vi "POST (Buffer).vi"(6 "timeout":i32=10000, 7 "output file":path, 8 "error in":errorcluster, 9 "buffer":string, 10 "url":string, 11 "session in":refnum<class "Session.lvclass">) -> (0 "error out":errorcluster, 1 "body":string, 2 "headers":string, 3 "session out":refnum<class "Session.lvclass">, 4 "status code":u32)   [LabVIEW 2019, in "NI_Advanced HTTP Client.lvlib" / "Session.lvclass"]
uses:
  Session.lvclass
  Session.lvclass/Session.ctl
  lvwebclient_32.dll
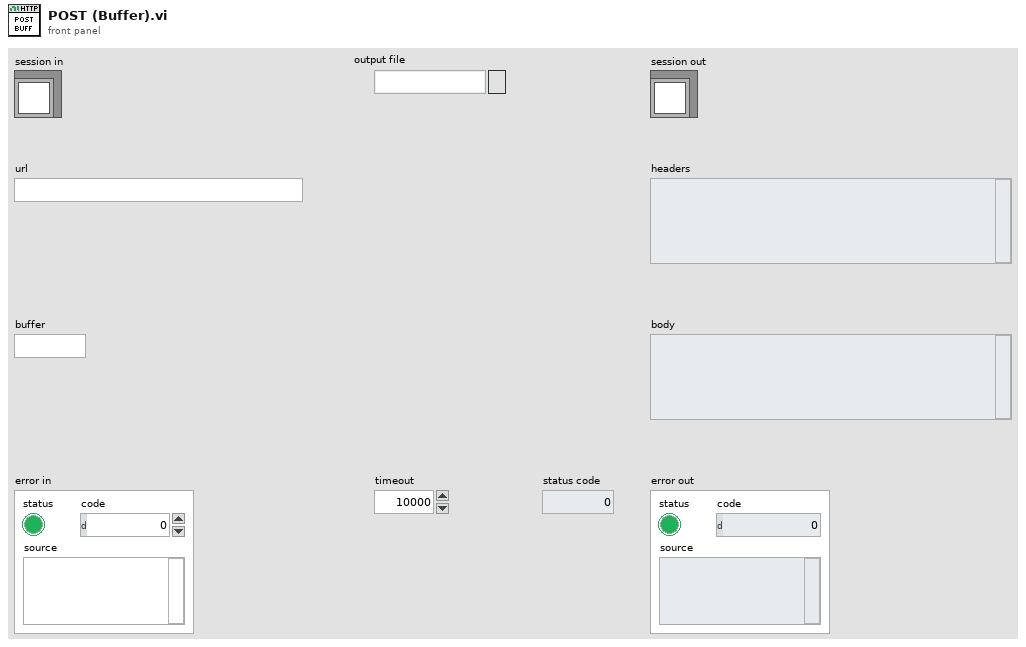
[diagram p1: front panel]
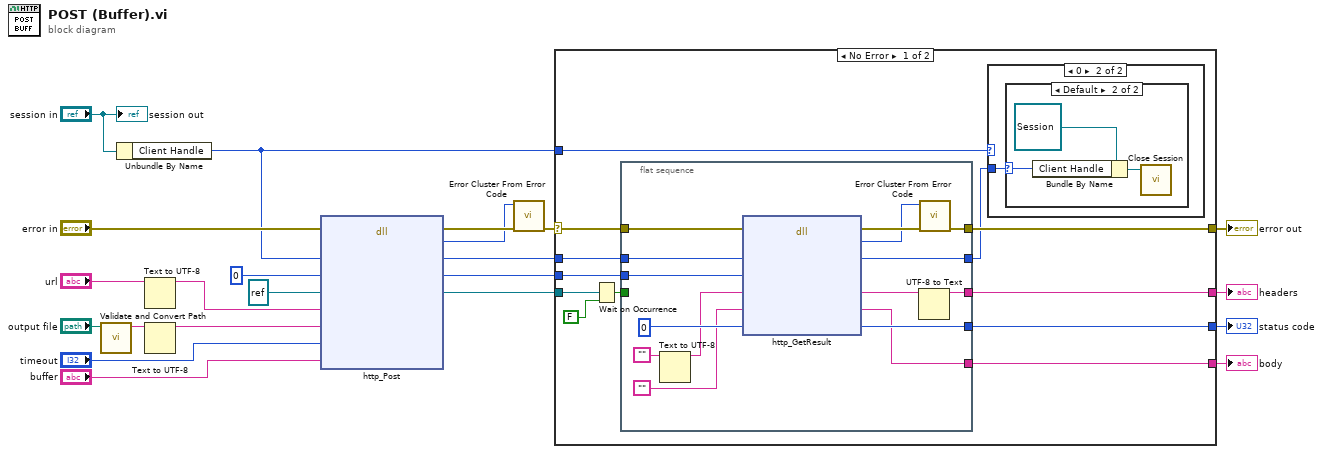
[diagram p0: block diagram]
diagram:
  n1 = call "Validate and Convert Path.vi"("path"="output file") -> ("validated path as string"=w14:string)  [unwired: 10 in]
  n2 = Unbundle By Name("session in") -> ("Client Handle"=w5:u32)
  n3 = Text to UTF-8(11:"url") -> (3:w3:string)  [unwired: 2 in, 1 out]
  n4 = Text to UTF-8(11:w14) -> (3:w2:string)  [unwired: 2 in, 1 out]
  n5 = dll-call lib="C:/Users/Localization Tester/Desktop/ni-adv-http-api/Advanced HTTP Client/lvwebclient_*.*" fn="http_Post"(error in="error in", "handle"=w5, "request"=u32 0, "completeOccurrence"=refnum<k4> refnum ("occurrence"), "url"=w3, "outPath"=w2, "timeout"="timeout", "postData"="buffer") -> (error out=w11:errorcluster, "return"=w10:i32, "handle"=w9:u32, "request"=w8:u32, "completeOccurrence"=w6:refnum<k4>)  [unwired: 6 in, 1 out]
  n6 = call <vilib>:"Error Cluster From Error Code.vi"("error in (no error)"=w11, "error code (0)"=w10) -> ("error out"=w22:errorcluster)  [unwired: 7 in]
  n7 = case shown="No Error" w22 {
    selector: w22 -> [w32 w54]
    tunnel: w6 -> [w34 _]
    tunnel: w9 -> [w31 _]
    tunnel: w8 -> [w30 _]
    tunnel: [w29 _] -> w19
    tunnel: [w28 _] -> w18
    tunnel: [w27 _] -> w17
    tunnel: [w26 w54] -> w16
    tunnel: w5 -> [w25 _]
    frame No Error {
      n8 = Wait on Occurrence(1:FALSE, 2:w34) -> (0:w33:bool)  [unwired: 1 in]
      n9 = flat-sequence {
        tunnel: w33 -> [_]
        tunnel: w32 -> [w53]
        tunnel: w31 -> [w52]
        tunnel: w30 -> [w51]
        tunnel: [w49] -> w29
        tunnel: [w44] -> w28
        tunnel: [w45] -> w27
        tunnel: [w43] -> w26
        tunnel: [w42] -> w24
        frame #0 {
          n10 = Text to UTF-8(11:"") -> (3:w40:string)  [unwired: 2 in, 1 out]
          n11 = dll-call lib="C:/Users/Localization Tester/Desktop/ni-adv-http-api/Advanced HTTP Client/lvwebclient_*.*" fn="http_GetResult"(error in=w53, "handle"=w52, "request"=w51, "returnHeader"=w40, "returnBody"="", "httpStatus"=u32 0) -> (error out=w48:errorcluster, "return"=w47:i32, "handle"=w42:u32, "returnHeader"=w46:string, "returnBody"=w45:string, "httpStatus"=w49:u32)  [unwired: 3 in, 1 out]
          n12 = UTF-8 to Text(11:w46) -> (3:w44:string)  [unwired: 2 in, 1 out]
          n13 = call <vilib>:"Error Cluster From Error Code.vi"("error in (no error)"=w48, "error code (0)"=w47) -> ("error out"=w43:errorcluster)  [unwired: 7 in]
        }
      }
      n14 = case shown="0" w25 {
        tunnel: w24 -> [_ w35]
        frame Default {
        }
        frame 0 {
          n15 = case shown="Default" w35 {
            selector: w35 -> [_ w38]
            frame 0 {
            }
            frame Default {
              n16 = Bundle By Name(cluster=refnum<class "Session.lvclass"> refnum ("NI_Advanced HTTP Client.lvlib:Session.lvclass"), "Client Handle"=w38) -> (w37:refnum<class "Session.lvclass">)
              n17 = call "Close Session.vi"("session"=w37) -> ()  [unwired: 10 in, 1 out]
            }
          }
        }
      }
    }
    frame Error {
    }
  }
  "error out" <- w16
  "headers" <- w18
  "body" <- w17
  "status code" <- w19
  "session out" <- "session in"
